vi "Translator.vi"(8 "error in (no error)":errorcluster, 11 "Input":variant) -> (0 "error out":errorcluster, 3 "Output":variant)   [LabVIEW 2014, in "TMRpcm.lvlib"]
doc: "An example of how to create the Translator to convert the LabVIEW VIs to Arduino C code."
uses:
  TMRpcm.lvlib
panel:
  out "Outputs":string[](array[string])
  out "Inputs":string[](array[string])
  out "Output Datatypes":string[](array[string])
  out "Input Datatypes":string[](array[string])
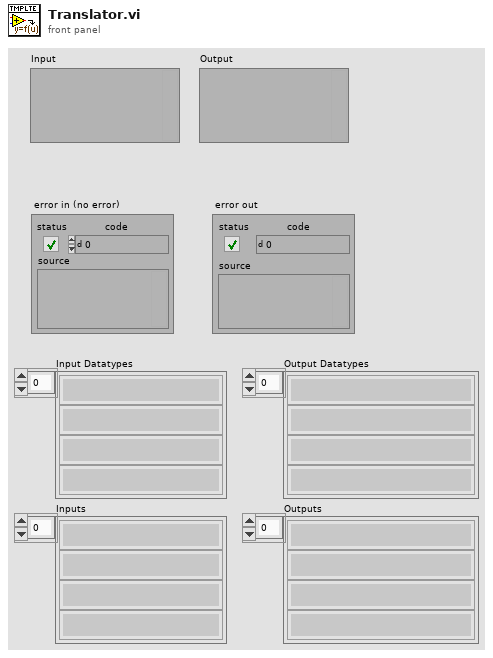
[diagram p1: front panel]
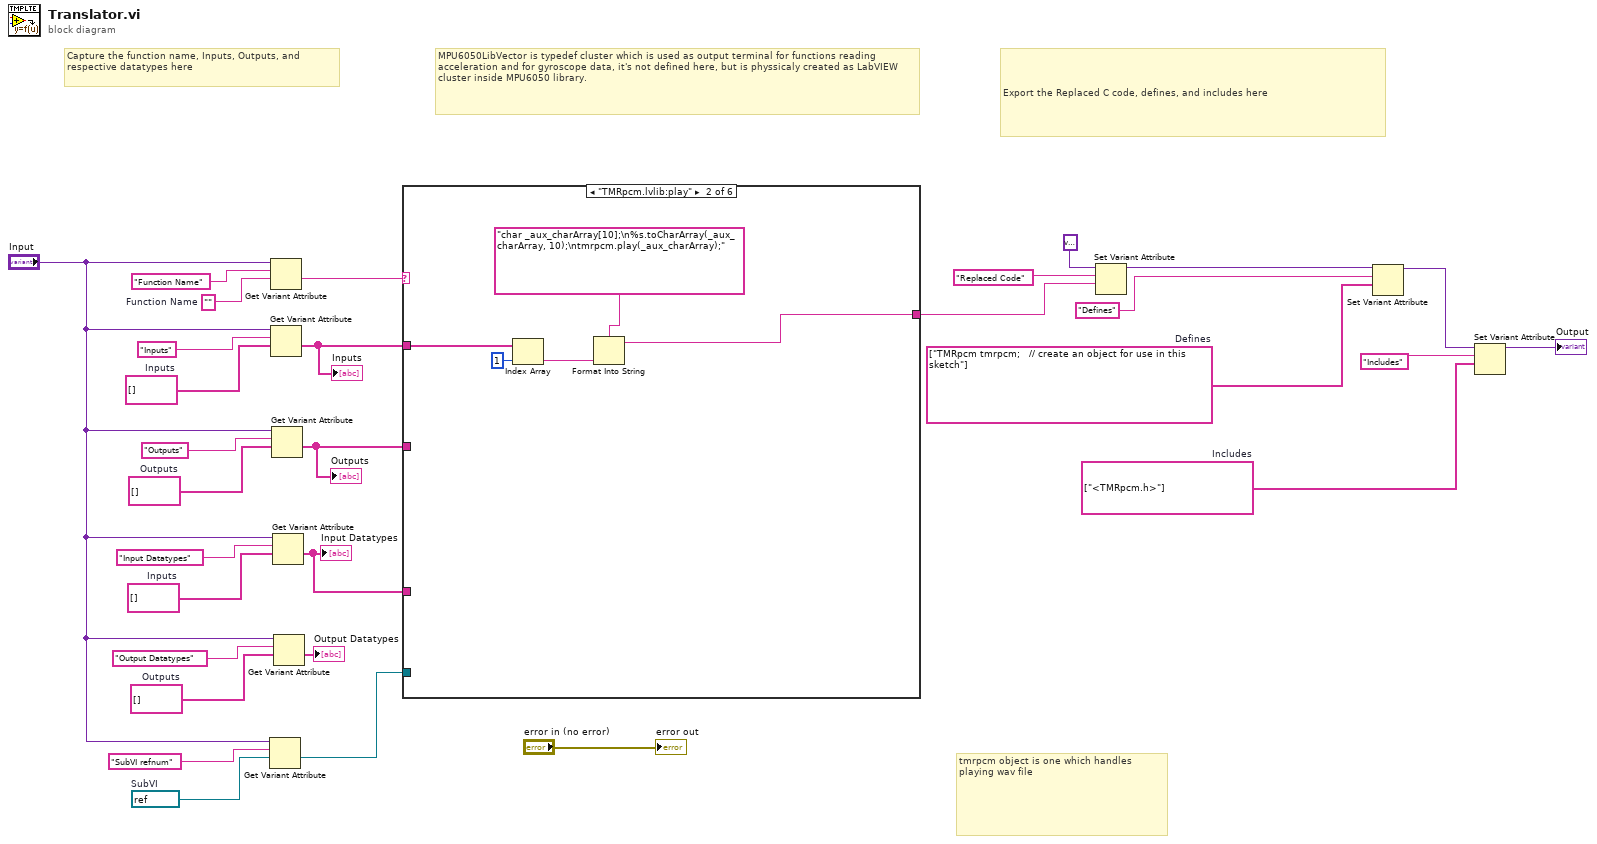
[diagram p0: block diagram]
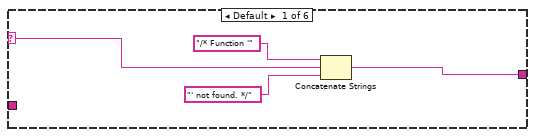
[diagram p2: hidden frame]
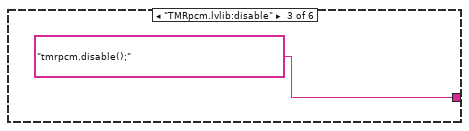
[diagram p3: hidden frame]
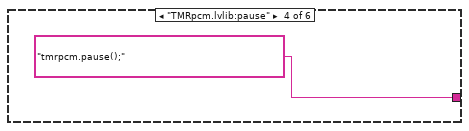
[diagram p4: hidden frame]
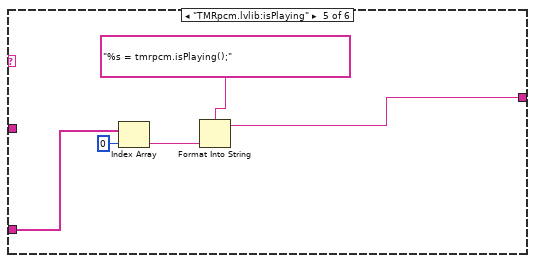
[diagram p5: hidden frame]
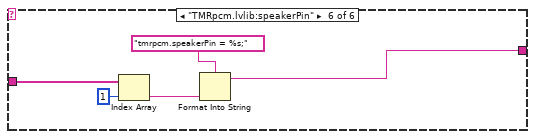
[diagram p6: hidden frame]
diagram:
  w2 = refnum<vi> refnum  # SubVI
  w6 = string[] ["TMRpcm tmrpcm;   // create an object for use in this sketch"]  # Defines
  w15 = string[] []  # Outputs
  w16 = string[] []  # Inputs
  w21 = string[] ["<TMRpcm.h>"]  # Includes
  w26 = string[] []  # Outputs
  w27 = string[] []  # Inputs
  w28 = ""  # Function Name
  # "MPU6050LibVector is typedef cluster which is used as output terminal for functions reading acceleration and for gyroscope data, it's not defined here, but is physsicaly created as LabVIEW cluster inside MPU6050 library."
  # "tmrpcm object is one which handles playing wav file"
  # "Capture the function name, Inputs, Outputs, and respective datatypes here"
  # "Export the Replaced C code, defines, and includes here"
  n1 = Get Variant Attribute(Variant="Input", name="SubVI refnum", default value (empty Variant)=w2) -> (value=w1:refnum<vi>)  [unwired: 1 in, 3 out]
  n2 = Get Variant Attribute(Variant="Input", name="Function Name", default value (empty Variant)=w28) -> (value=w23:string)  [unwired: 1 in, 3 out]
  n3 = Get Variant Attribute(Variant="Input", name="Inputs", default value (empty Variant)=w27) -> (value=w11:string[])  [unwired: 1 in, 3 out]
  "Inputs" <- w11
  n4 = Get Variant Attribute(Variant="Input", name="Outputs", default value (empty Variant)=w26) -> (value=w12:string[])  [unwired: 1 in, 3 out]
  "Outputs" <- w12
  n5 = Get Variant Attribute(Variant="Input", name="Input Datatypes", default value (empty Variant)=w16) -> (value=w5:string[])  [unwired: 1 in, 3 out]
  "Input Datatypes" <- w5
  n6 = Get Variant Attribute(Variant="Input", name="Output Datatypes", default value (empty Variant)=w15) -> (value=→"Output Datatypes":string[])  [unwired: 1 in, 3 out]
  n7 = case shown="\"TMRpcm.lvlib:play\"" w23 {
    selector: w23 -> [w33 _ _ _ _ _]
    tunnel: [w31 w36 "tmrpcm.disable();" ("format string") "tmrpcm.pause();" ("format string") w44 w48] -> w22
    tunnel: w11 -> [_ w39 _ _ _ w51]
    tunnel: w12 -> [_ _ _ _ w42 _]
    tunnel: w5 -> [_ _ _ _ _ _]
    tunnel: w1 -> [_ _ _ _ _ _]
    frame Default {
      n8 = Concatenate Strings("/* Function '", w33, "' not found. */") -> (w31:string)
    }
    frame "TMRpcm.lvlib:play" {
      n9 = Index Array(array=w39, index=1) -> (element=w37:string)
      n10 = Format Into String(format string="char _aux_charArray[10];\n%s.toCharArray(_aux_charArray, 10);\ntmrpcm.play(_aux_charArray);", w37) -> (resulting string=w36:string)  [unwired: 2 in, 1 out]
    }
    frame "TMRpcm.lvlib:disable" {
    }
    frame "TMRpcm.lvlib:pause" {
    }
    frame "TMRpcm.lvlib:isPlaying" {
      n11 = Index Array(array=w42, index=0) -> (element=w45:string)
      n12 = Format Into String(format string="%s = tmrpcm.isPlaying();", w45) -> (resulting string=w44:string)  [unwired: 2 in, 1 out]
    }
    frame "TMRpcm.lvlib:speakerPin" {
      n13 = Index Array(array=w51, index=1) -> (element=w49:string)
      n14 = Format Into String(format string="tmrpcm.speakerPin = %s;", w49) -> (resulting string=w48:string)  [unwired: 2 in, 1 out]
    }
  }
  n15 = Set Variant Attribute(Variant=variant ("variant"), name="Replaced Code", value=w22) -> (Variant out=w9:variant)  [unwired: 1 in, 2 out]
  n16 = Set Variant Attribute(Variant=w9, name="Defines", value=w6) -> (Variant out=w8:variant)  [unwired: 1 in, 2 out]
  n17 = Set Variant Attribute(Variant=w8, name="Includes", value=w21) -> (Variant out=→"Output":variant)  [unwired: 1 in, 2 out]
  "error out" <- "error in (no error)"
